vi "Create RIO APU Mapping.vi"(8 "error in (no error)":errorcluster, 9 "APUs":string[](array[string]), 10 "rio name":string, 11 "Section Ptr":T1 format="%.0x") -> (0 "error out":errorcluster, 1 "APUs":string[](array[string]), 3 "Section Ptr":T1 format="%.0x")   [LabVIEW 2015, in "Engine Simulation Toolkit System Explorer.lvlib"]
uses:
  Engine Simulation Toolkit System Explorer.lvlib
  <vilib>/NI Veristand/Custom Device API/Custom Device Item Ref.ctl
  <vilib>/NI Veristand/Custom Device API/Set Item Property (String Array).vi
  <vilib>/NI Veristand/Custom Device API/Custom Device API.lvlib
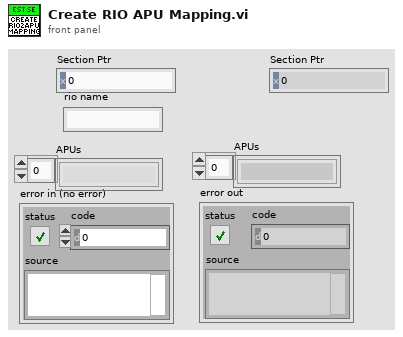
[diagram p1: front panel]
types:
  T1 = typedef "Custom Device API.lvlib/Custom Device Item Ref.ctl" = u64
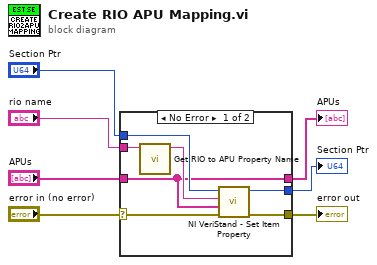
[diagram p0: block diagram]
diagram:
  n1 = case shown="No Error" "error in (no error)" {
    selector: "error in (no error)" -> [w10 w17]
    tunnel: [w9 w17] -> w6
    tunnel: "Section Ptr" -> [w14 w16]
    tunnel: [w13 w16] -> w4
    tunnel: "rio name" -> [w12 _]
    tunnel: "APUs" -> [w8 w15]
    tunnel: [w8 w15] -> w1
    frame No Error {
      n2 = call "Get RIO to APU Property Name.vi"("rio name"=w12) -> ("property name"=w11:string)  [unwired: 10 in]
      n3 = call-poly <vilib>:"NI VeriStand - Set Item Property.vi"("error in (no error)"=w10, "Value"=w8, "Property Name"=w11, "Item Ref in"=w14) -> ("error out"=w9:errorcluster, "Item Ref out"=w13:T1)  [unwired: 5 in, 1 out]
    }
    frame Error {
    }
  }
  "error out" <- w6
  "Section Ptr" <- w4
  "APUs" <- w1
